vi "Read Test Executive Ref.vi"(11 "ITest Executive Builder Dialog in":refnum<class "ITest Executive Builder Dialog.lvclass">) -> (3 "ITest Executive Builder Dialog out":refnum<class "ITest Executive Builder Dialog.lvclass">, 4 "Test Executive Ref":refnum<data-value>)   [LabVIEW 2017, in "ITest Executive Builder Dialog.lvclass"]
uses:
  ITest Executive Builder Dialog.lvclass
  <vilib>/gpm_packages/@cs/test-executive/Source/Test Executive/ITestExecutive/ITest Executive.lvclass
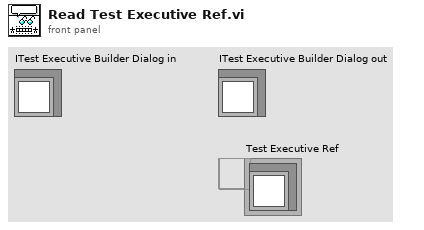
[diagram p1: front panel]
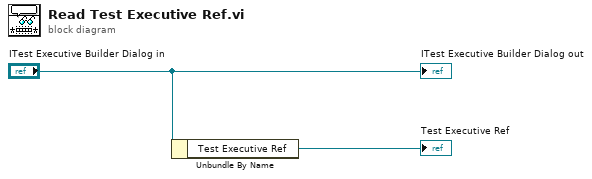
[diagram p0: block diagram]
diagram:
  n1 = Unbundle By Name("ITest Executive Builder Dialog in") -> ("Test Executive Ref"=→"Test Executive Ref":refnum<data-value>)
  "ITest Executive Builder Dialog out" <- "ITest Executive Builder Dialog in"
